vi "CaseStructure Format FrameNames Into C code Strings.vi"(11 "FrameNames in":string[](array[string])) -> (3 "c code cases names":string[](array[string]))   [LabVIEW 2014]
doc: "Takes CaseStructure FrameNames and returns names suitable for switch(){case \"someName\": }, replace whitespaces with underscore:\nsome name ---> some_name"
uses:
  <vilib>/regexp/Match Regular Expression.xnode
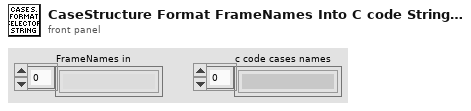
[diagram p1: front panel]
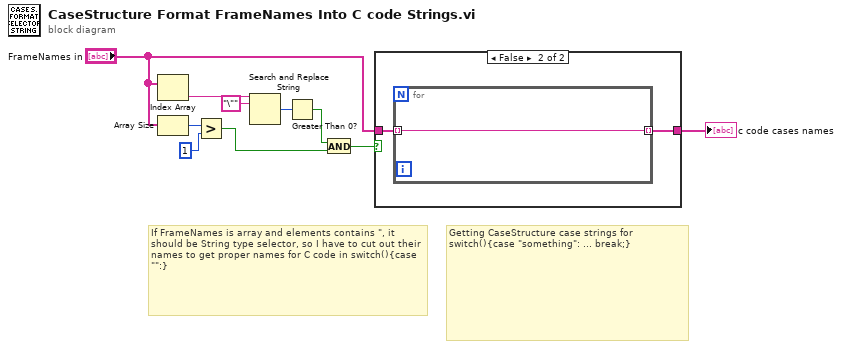
[diagram p0: block diagram]
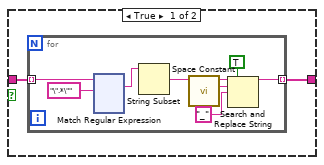
[diagram p2: hidden frame]
diagram:
  # "Getting CaseStructure case strings for switch(){case \"something\": ... break;}"
  # "If FrameNames is array and elements contains \", it should be String type selector, so I have to cut out their names to get proper names for C code in switch(){case \"\":}"
  n1 = Index Array(array="FrameNames in") -> (element=w3:string)  [unwired: 1 in]
  n2 = Array Size(array="FrameNames in") -> (size(s)=w1:i32)
  n3 = Greater?(x=w1, y=1) -> (0:w7:bool)
  n4 = Search and Replace String(input string=w3, search string="\"") -> (number of replacements=w5:i32)  [unwired: 6 in, 3 out]
  n5 = Greater Than 0?(x=w5) -> (x > 0?=w6:bool)
  n6 = And(x=w6, y=w7) -> (x .and. y?=w8:bool)
  n7 = case shown="False" w8 {
    tunnel: "FrameNames in" -> [w12 w136]
    tunnel: [w11 w135] -> w10
    frame True {
      n8 = for {
        tunnel: w12 -> [w20] mode=indexing
        tunnel: [w13] -> w11 mode=indexing
        n9 = xnode "Match Regular Expression"("input string"=w20, "regular expression"="\".*\"") -> ("whole match"=w18:string)  [unwired: 4 in, 4 out]
        n10 = String Subset(string=w18) -> (substring=w17:string)  [unwired: 2 in]
        n11 = call <vilib>:"Space Constant.vi"() -> ("String"=w16:string)
        n12 = Search and Replace String(replace all?=TRUE ("replace all? (F)"), input string=w17, search string=w16, replace string="_" ("replace string (\"\")")) -> (result string=w13:string)  [unwired: 4 in, 3 out]
      }
    }
    frame False {
      n13 = for {
        tunnel: w136 -> [w137] mode=indexing
        tunnel: [w137] -> w135 mode=indexing
      }
    }
  }
  "c code cases names" <- w10
